vi "Set voltage and current.vi"(4 "OverCurrent Protection (F:Off)":bool, 5 "Output Current (A) (0.0)":dbl min=0.0 max=3.0 step=0.001 format="%.3f", 6 "OVP(V) (0.000)":dbl min=0.0 max=38.5 step=0.01 format="%.3f", 7 "Output Voltage (V) (0.0)":dbl min=0.0 max=36.0 step=0.01 format="%.3f", 8 "error in (no error)":errorcluster, 9 "Output State (F:Off)":bool, 10 "Channel Select (1)":u8=1 min=1 max=3, 11 "VISA session":refnum<visa-resource-name>) -> (0 "error out":errorcluster, 1 "Actual Output Current (A)":dbl format="%.3f", 2 "Actual Output Voltage(V)":dbl format="%.3f", 3 "dup VISA session":refnum<visa-resource-name>)   [LabVIEW 2010]
doc: "This VI uses various subVI's to configure the instrument and read back a measurement."
panel:
  # "PROGRAMMABLE POWER SUPPLY PST3201 PST3202 PSS3203"
  # "ON\nOFF"
  # "OFF"
  # "ON"
  # "WARNINGS: \nRS232 message terminators: AS there is no signal of end message on RS232 bus, therefore, use LF as \nmessage terminator. When a series of commands are sent to the instrument, it must add a LF to be a\njudhment for message terminator. As for query command, the return message of the instrument is also\nadded a LF for PC to judge message terminator."
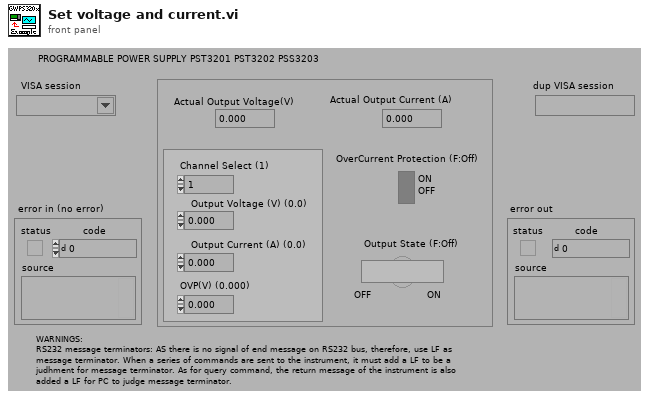
[diagram p1: front panel]
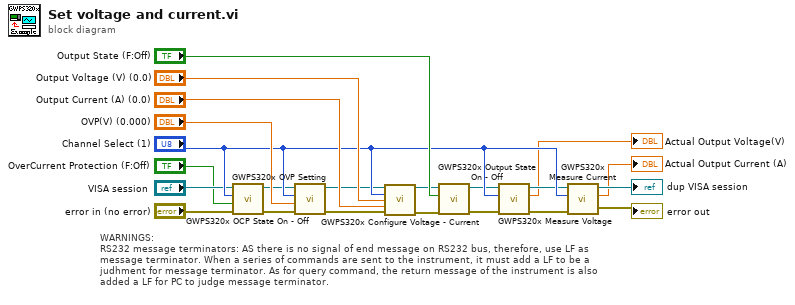
[diagram p0: block diagram]
diagram:
  # "WARNINGS: \nRS232 message terminators: AS there is no signal of end message on RS232 bus, therefore, use LF as \nmessage terminator. When a series of commands are sent to the instrument, it must add a LF to be a\njudhment for message terminator. As for query command, the return message of the instrument is also\nadded a LF for PC to judge message terminator."
  n1 = call <instrlib>:"GWPS320x OCP State On - Off.vi"("error in (no error)"="error in (no error)", "OverCurrent Protection (T:Off)"="OverCurrent Protection (F:Off)", "Channel Select (1)"="Channel Select (1)", "VISA session"="VISA session") -> ("error out"=w7:errorcluster, "dup VISA session"=w8:refnum<visa-resource-name>)  [unwired: 6 in]
  n2 = call <instrlib>:"GWPS320x OVP Setting.vi"("error in (no error)"=w7, "OVP(V) (0.000)"="OVP(V) (0.000)", "Channel Select (1)"="Channel Select (1)", "VISA session"=w8) -> ("error out"=w9:errorcluster, "dup VISA session"=w10:refnum<visa-resource-name>)  [unwired: 6 in]
  n3 = call <instrlib>:"GWPS320x Configure Voltage - Current.vi"("VISA session"=w10, "Channel Select (1)"="Channel Select (1)", "Output Voltage (V) (0.0)"="Output Voltage (V) (0.0)", "Output Current (A) (0.0)"="Output Current (A) (0.0)", "error in (no error)"=w9) -> ("dup VISA session"=w12:refnum<visa-resource-name>, "error out"=w11:errorcluster)  [unwired: 9 in]
  n4 = call <instrlib>:"GWPS320x Output State On - Off.vi"("error in (no error)"=w11, "Output State (F:Off)"="Output State (F:Off)", "VISA session"=w12) -> ("error out"=w13:errorcluster, "dup VISA session"=w14:refnum<visa-resource-name>)  [unwired: 7 in]
  n5 = call <instrlib>:"GWPS320x Measure Voltage.vi"("error in (no error)"=w13, "Channel Select (1)"="Channel Select (1)", "VISA session"=w14) -> ("error out"=w5:errorcluster, "Actual Output Voltage(V)"=→"Actual Output Voltage(V)":dbl, "dup VISA session"=w6:refnum<visa-resource-name>)  [unwired: 6 in]
  n6 = call <instrlib>:"GWPS320x Measure Current.vi"("error in (no error)"=w5, "Channel Select (1)"="Channel Select (1)", "VISA session"=w6) -> ("error out"=→"error out":errorcluster, "Actual Output Current (A)"=→"Actual Output Current (A)":dbl, "dup VISA session"=→"dup VISA session":refnum<visa-resource-name>)  [unwired: 6 in]
